vi "Handle Data.vi"(8 "error in (no error)":errorcluster, 10 "Data":dbl, 11 "DataHandler in":refnum<class "DataHandler.lvclass">) -> (0 "error out":errorcluster, 3 "DataHandler out":refnum<class "DataHandler.lvclass">)   [LabVIEW 2020, in "LAF2024Q2.lvlib" / "DataHandler.lvclass"]
uses:
  DataHandler.lvclass
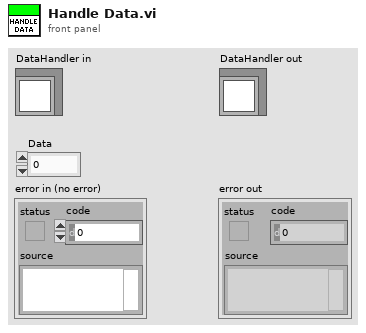
[diagram p1: front panel]
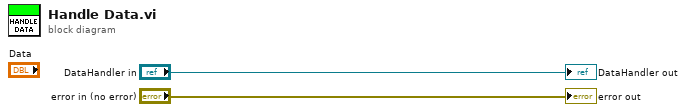
[diagram p0: block diagram]
diagram:
  "error out" <- "error in (no error)"
  "DataHandler out" <- "DataHandler in"
